vi "registro-usuario-v1.vi"() -> ()   [LabVIEW 2024]
uses:
  <vilib>/Utility/file.llb/Write Delimited Spreadsheet (string).vi
panel:
  in  "stop":bool
  in  "registrButt":bool
  in  "Registrar Usuario":T1
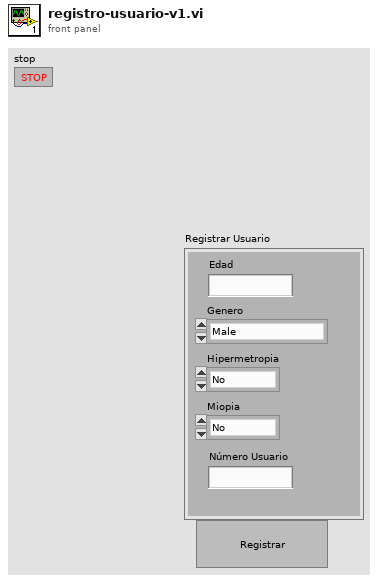
[diagram p1: front panel]
types:
  T1 = cluster{"Número Usuario":string, "Edad":string, "Genero":enum16{"Male", "Female"}, "Hipermetropia":enum16{"No", "Si"}, "Miopia":enum16{"No", "Si"}}
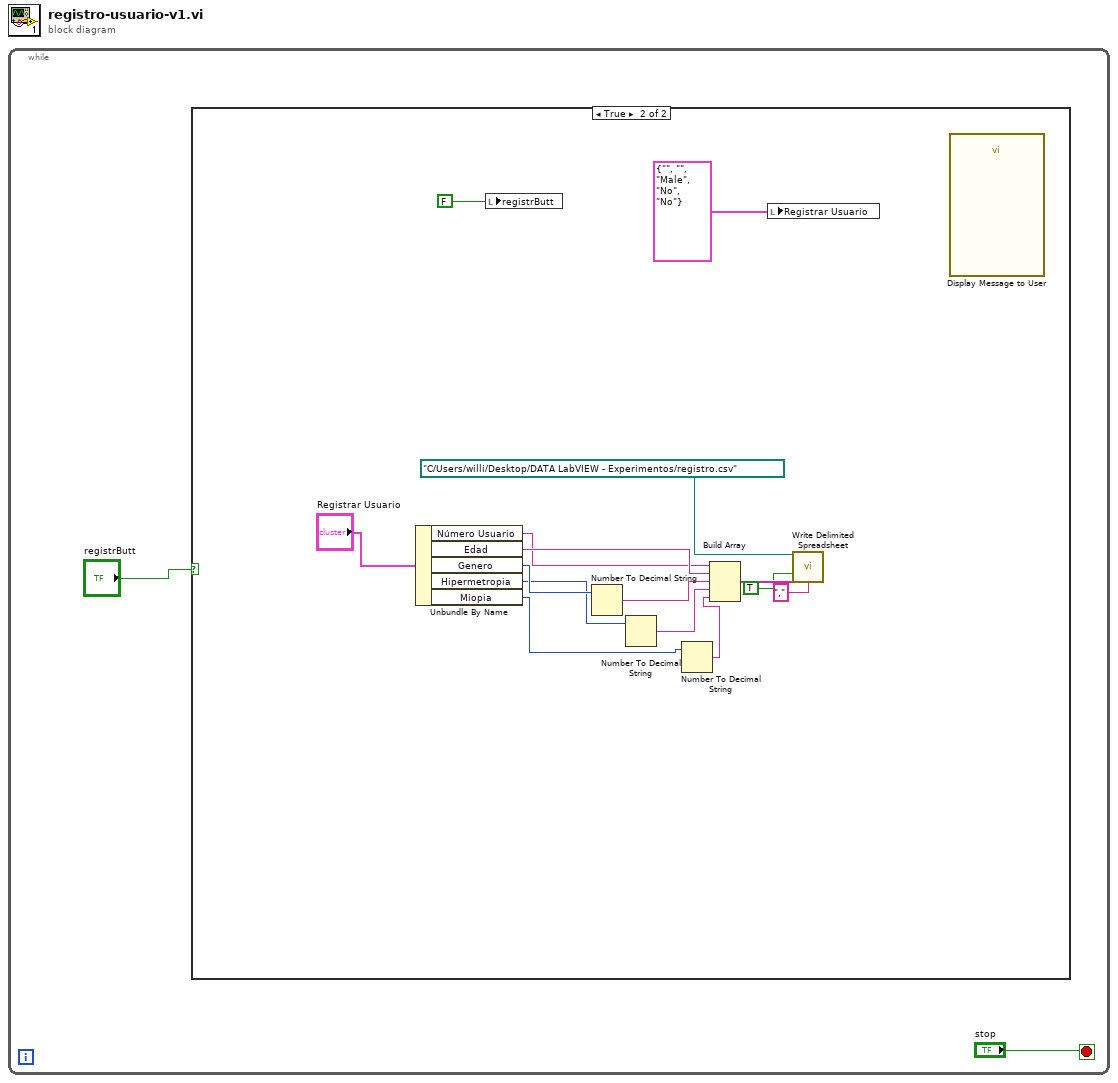
[diagram p0: block diagram]
diagram:
  n1 = while {
    stop <- "stop" stop-if-true
    n2 = case shown="True" "registrButt" {
      frame False {
      }
      frame True {
        n3 = Unbundle By Name("Registrar Usuario") -> ("Número Usuario"=w3:string, "Edad"=w4:string, "Genero"=w7:enum16{"Male", "Female"}, "Hipermetropia"=w6:enum16{"No", "Si"}, "Miopia"=w5:enum16{"No", "Si"})
        n4 = local write "registrButt"(FALSE) -> ()
        n5 = Number To Decimal String(number=w7) -> (decimal integer string=w8:string)  [unwired: 1 in]
        n6 = Number To Decimal String(number=w6) -> (decimal integer string=w9:string)  [unwired: 1 in]
        n7 = Number To Decimal String(number=w5) -> (decimal integer string=w12:string)  [unwired: 1 in]
        n8 = Build Array(w3, w4, w8, w9, w12) -> (w16:string[])
        n9 = local write "Registrar Usuario"(T1 {"Número Usuario"="", "Edad"="", "Genero"=enum."Male", "Hipermetropia"=enum."No", "Miopia"=enum."No"} ("Registrar Usuario")) -> ()
        n10 = call-poly <vilib>:"Write Delimited Spreadsheet.vi"("file path (dialog if empty)"=path "C:/Users/willi/Desktop/DATA LabVIEW - Experimentos/registro.csv", "1D data"=w16, "append to file? (new file:F)"=TRUE, "delimiter (\\t)"="," ("delimiter (\\t)")) -> ()  [unwired: 10 in, 2 out]
        n11 = call "Display Message to User"() -> ()  [unwired: 10 in, 2 out]
      }
    }
  }
